vi "Read Control Experiment.vi"(8 "error in (no error)":errorcluster, 11 "SweepControl in":refnum<class "SMO.SweepControl.lvclass">) -> (0 "error out":errorcluster, 2 "Control Experiment.lvclass":refnum<class "Control Experiment.lvclass">, 3 "SweepControl out":refnum<class "SMO.SweepControl.lvclass">)   [LabVIEW 2019, in "SMO.SweepControl.lvclass"]
uses:
  SMO.SweepControl.lvclass
  Control Experiment/Control Experiment.lvclass
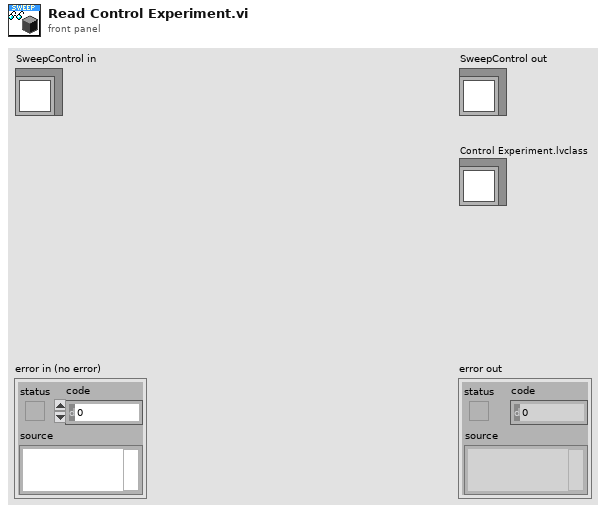
[diagram p1: front panel]
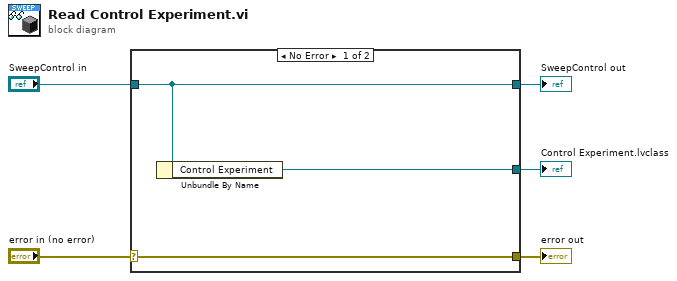
[diagram p0: block diagram]
diagram:
  n1 = case shown="No Error" "error in (no error)" {
    selector: "error in (no error)" -> [w8 w9]
    tunnel: [w8 w9] -> w4
    tunnel: [w7 w10] -> w2
    tunnel: "SweepControl in" -> [w7 w10]
    tunnel: [w6 _] -> w1
    frame No Error {
      n2 = Unbundle By Name(w7) -> ("Control Experiment"=w6:refnum<class "Control Experiment.lvclass">)
    }
    frame Error {
    }
  }
  "error out" <- w4
  "SweepControl out" <- w2
  "Control Experiment.lvclass" <- w1
